vi "CSM - Wait for All Modules to Exit.vi"(6 "Wait (5000 ms)":u32=5000, 8 "Error In":errorcluster caption="error in (no error)", 11 "CSM Names":string[](array[string])) -> (0 "error out":errorcluster, 1 "Waited (ms)":u32, 2 "CSMs Left":string[](array[string]))   [LabVIEW 2017, in "Communicable State Machine.lvlib"]
doc: "### CSM - Wait for All Modules to Exit.vi\n\nWait for a group of CSM modules to go offline within the specified timeout period, usually used for program exit.\n\n-- <b>Controls</b> --\n- <b>CSM Names</b>: CSM module names\n- <b>Timeout(5000ms)</b>: Wait timeout, default is 5s\n\n-- <b>Indicators</b> --\n- <b>CSMs Left</b>: CSM modules that did not go offline within the timeout period\n- <b>Waited(ms)</b>: Time waited"
uses:
  Communicable State Machine.lvlib
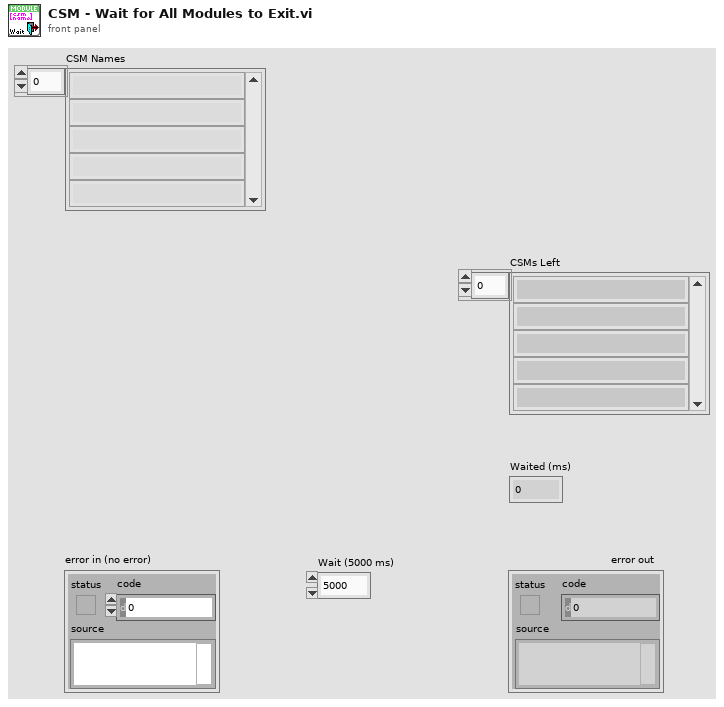
[diagram p1: front panel]
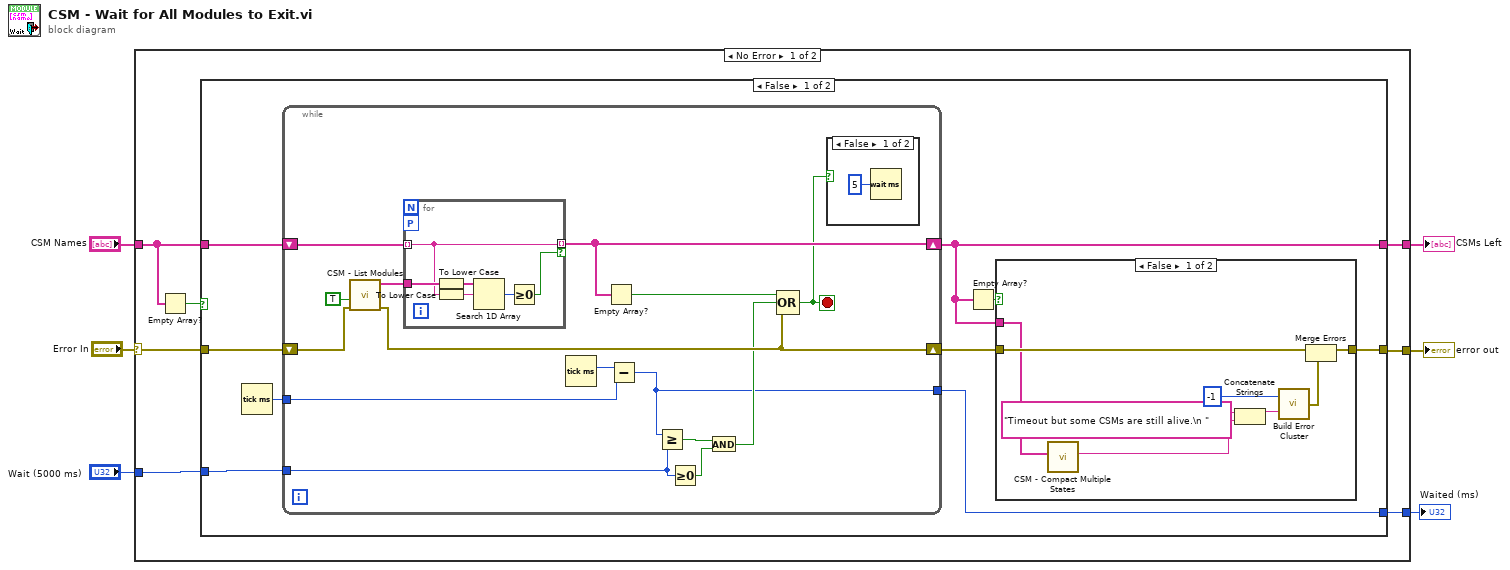
[diagram p0: block diagram]
diagram:
  n1 = case shown="No Error" "Error In" {
    selector: "Error In" -> [w13 w57]
    tunnel: [w11 w57] -> w5
    tunnel: "CSM Names" -> [w8 w56]
    tunnel: [w10 w56] -> w3
    tunnel: "Wait (5000 ms)" -> [w12 _]
    tunnel: [w7 _] -> w1
    frame No Error {
      n2 = Empty Array?(array=w8) -> (empty?=w9:bool)
      n3 = case shown="False" w9 {
        tunnel: w8 -> [w22 w55]
        tunnel: w13 -> [w21 w54]
        tunnel: w12 -> [w19 _]
        tunnel: [w17 w54] -> w11
        tunnel: [w15 w55] -> w10
        tunnel: [w14 _] -> w7
        frame False {
          n4 = Tick Count (ms)() -> (millisecond timer value=w20:u32)
          n5 = while {
            shift-right: [w43] -> w15
            shift-left: w22 -> [w45]
            shift-right: [w40] -> w16
            shift-left: w21 -> [w42]
            tunnel: w20 -> [w39]
            tunnel: w19 -> [w33]
            tunnel: [w32] -> w14
            stop <- w38 stop-if-true
            n6 = call "CSM - List Modules.vi"("Error In"=w42, "With Instance? (F)"=TRUE ("All?")) -> ("error out"=w40:errorcluster, "Module Names"=w44:string[])  [unwired: 8 in]
            n7 = for {
              tunnel: w45 -> [w52] mode=indexing
              tunnel: w44 -> [w53]
              tunnel: [w52] -> w43 mode=indexing if=w51
              workers-P: _ -> [_]
              n8 = To Lower Case(string=w53) -> (all lower case string=w48:string[])
              n9 = To Lower Case(string=w52) -> (all lower case string=w49:string)
              n10 = Search 1D Array(1D array=w48, element=w49) -> (index of element=w50:i32)  [unwired: 1 in]
              n11 = Greater Or Equal To 0?(x=w50) -> (x >= 0?=w51:bool)
            }
            n12 = Tick Count (ms)() -> (millisecond timer value=w37:u32)
            n13 = Empty Array?(array=w43) -> (empty?=w41:bool)
            n14 = Subtract(x=w37, y=w39) -> (x-y=w32:u32)
            n15 = Greater Or Equal?(x=w32, y=w33) -> (x >= y?=w36:bool)
            n16 = Greater Or Equal To 0?(x=w33) -> (x >= 0?=w35:bool)
            n17 = And(x=w36, y=w35) -> (x .and. y?=w34:bool)
            n18 = Compound Arithmetic op=OR(w41, w34, w40) -> (w38:bool)
            n19 = case shown="False" w38 {
              frame False {
                n20 = Wait (ms)(milliseconds to wait=u32 5) -> ()  [unwired: 1 out]
              }
              frame True {
              }
            }
          }
          n21 = Empty Array?(array=w15) -> (empty?=w18:bool)
          n22 = case shown="False" w18 {
            tunnel: [w29 w31] -> w17
            tunnel: w16 -> [w30 w31]
            tunnel: w15 -> [w24 _]
            frame False {
              n23 = call "CSM - Compact Multiple States.vi"("Multiple States"=w24) -> ("States"=w23:string)  [unwired: 9 in]
              n24 = Concatenate Strings("Timeout but some CSMs are still alive.\n " ("String to Prepend to source (\"\")"), w23) -> (w25:string)
              n25 = call "Build Error Cluster.vi"("String to Prepend to Source (\"\")"=w25, "Code"=-1 ("code")) -> ("error out"=w28:errorcluster)
              n26 = Merge Errors(w30, w28) -> (w29:errorcluster)
            }
            frame True {
            }
          }
        }
        frame True {
        }
      }
    }
    frame Error {
    }
  }
  "error out" <- w5
  "CSMs Left" <- w3
  "Waited (ms)" <- w1
